vi "Seperate at Decimal Point.vi"(11 "Rotations":dbl) -> (2 "Rotations":dbl, 3 "Angle":T1 scale format="%.3f")   [LabVIEW 2023, in "Thor-SwerveDrive_ACT.lvlib"]
uses:
  Thor-SwerveDrive_ACT.lvlib
  Shared Code/TypeDefs/Dial_Compase heading unit circle CCW positive.ctl
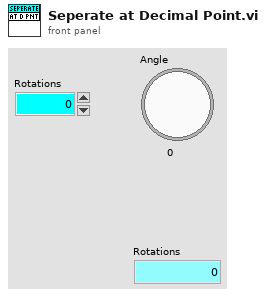
[diagram p1: front panel]
types:
  T1 = typedef "Dial_Compase heading unit circle CCW positive.ctl" = dbl
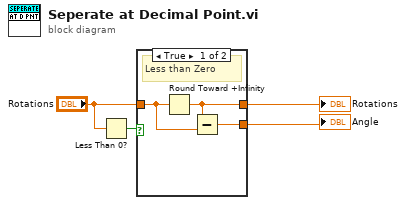
[diagram p0: block diagram]
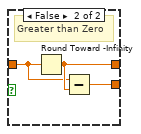
[diagram p2: hidden frame]
diagram:
  n1 = Less Than 0?(x="Rotations") -> (x < 0?=w4:bool)
  n2 = case shown="True" w4 {
    tunnel: "Rotations" -> [w6 w9]
    tunnel: [w7 w10] -> w2
    tunnel: [w5 w8] -> w1
    frame True {
      # "Less than Zero"
      n3 = Round Toward +Infinity(x=w6) -> (ceil(x): smallest int >= x=w7:dbl)
      n4 = Subtract(x=w7, y=w6) -> (x-y=w5:dbl)
    }
    frame False {
      # "Greater than Zero"
      n5 = Round Toward -Infinity(1:w9) -> (0:w10:dbl)
      n6 = Subtract(x=w9, y=w10) -> (x-y=w8:dbl)
    }
  }
  "Angle" <- w1
  "Rotations" <- w2
